vi "elevador.vi"() -> ()   [LabVIEW 2018]
panel:
  out "Porta aberta":bool
  in  "Door":enum32{"0", "1"}(radio)
  in  "Select":enum32{"0", "1", "2"}(radio)
  out "Andar":dbl
  out "RC floor":bool
  out "1 floor":bool
  out "2 floor":bool
  in  "stop":bool
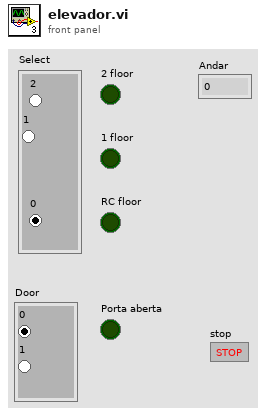
[diagram p1: front panel]
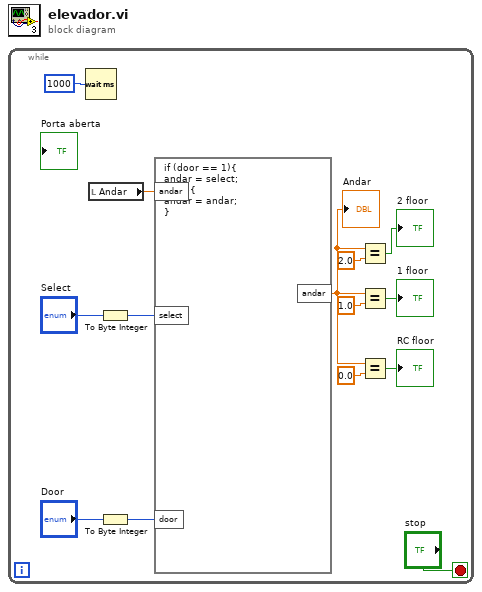
[diagram p0: block diagram]
diagram:
  n1 = while {
    stop <- "stop" stop-if-true
    n2 = Wait (ms)(milliseconds to wait=u32 1000) -> ()  [unwired: 1 out]
    n3 = local read "Andar"() -> (w9:dbl)
    n4 = To Byte Integer(number="Select") -> (8bit integer=w12:i8)
    n5 = To Byte Integer(number="Door") -> (8bit integer=w10:i8)
    n6 = formula code="if (door == 1){\nandar = select;\n}else{\nandar = andar;\n}"("select"=w12, "door"=w10, "andar"=w9) -> ("andar"=w7:dbl)
    "Andar" <- w7
    n7 = Equal?(x=w7, y=2.0) -> (x = y?=→"2 floor":bool)
    n8 = Equal?(x=w7, y=1.0) -> (x = y?=→"1 floor":bool)
    n9 = Equal?(x=w7, y=0.0) -> (x = y?=→"RC floor":bool)
  }
